vi "Insert DateTime Into Path.vi"(11 "File":path) -> (3 "appended path":path)   [LabVIEW 2020, in "Log.lvclass"]
uses:
  Log.lvclass
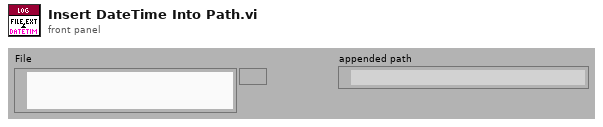
[diagram p1: front panel]
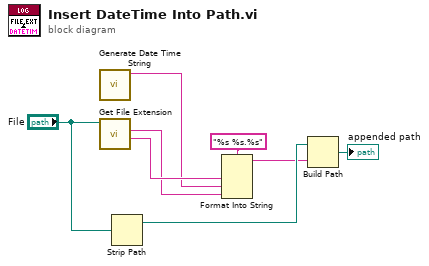
[diagram p0: block diagram]
diagram:
  n1 = call "Generate Date Time String.vi"() -> ("Date time string"=w1:string)  [unwired: 10 in, 1 out]
  n2 = call <vilib>:"Get File Extension.vi"("file"="File") -> ("filename without extension"=w7:string, "lowercase file extension"=w6:string)  [unwired: 1 in, 8 out]
  n3 = Strip Path(path="File") -> (stripped path=w5:path)  [unwired: 1 out]
  n4 = Format Into String(format string="%s %s.%s", w7, w1, w6) -> (resulting string=w4:string)  [unwired: 2 in, 1 out]
  n5 = Build Path(base path=w5, name or relative path=w4) -> (appended path=→"appended path":path)
